vi "Configure Program Mode.vi"(0 "VISA resource name":refnum<visa-resource-name>, 1 "Voltage Low Limit (0 V)":dbl min=0.0 max=400.0 format="%.1f", 2 "Voltage High Limit (300 V)":dbl=300.0 min=0.0 max=400.0 format="%.1f", 3 "Single Step Mode (F:Disable)":bool, 5 "Loop Cycle (1)":i32=1 min=0 max=9999 step=1, 7 "Start Angle (0)":i32 min=0 max=359, 9 "End Angle: (0)":i32 min=0 max=359, 11 "error in (no error)":errorcluster, 12 "Frequency Low Limit (40 Hz)":dbl=45.0 min=0.0 max=500.0 format="%.1f", 13 "Frequency High Limit (500 Hz)":dbl=500.0 min=0.0 max=500.0 format="%.1f", 14 "Enable Over Current Fold Back (F:Disable)":bool) -> (4 "VISA resource name out":refnum<visa-resource-name>, 15 "error out":errorcluster)   [LabVIEW 2014, in "eec 6700.lvlib"]
doc: "Sets the instrument in program mode and configures the parameters in it.\n\nIn the program mode the instrument can be programmed for a sequence of operations/Settings with the help of a list of 50 sequential memories with 9 steps each. Each step can be configured with user configurable testing parameters such as test time, high and low limits, etc."
uses:
  <instrlib>/eec 6700/eec 6700.lvlib
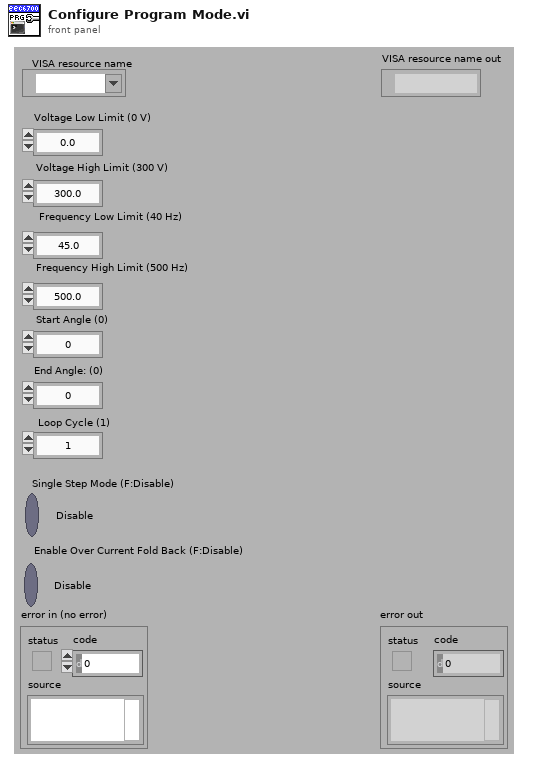
[diagram p1: front panel]
types:
  T1 = typedef "eec 6700.lvlib/Extended User Data.ctl" = cluster{"Firmware Version":string, "eec Models":enum16{"6605", "6610", "6620", "6630", "6650"}}
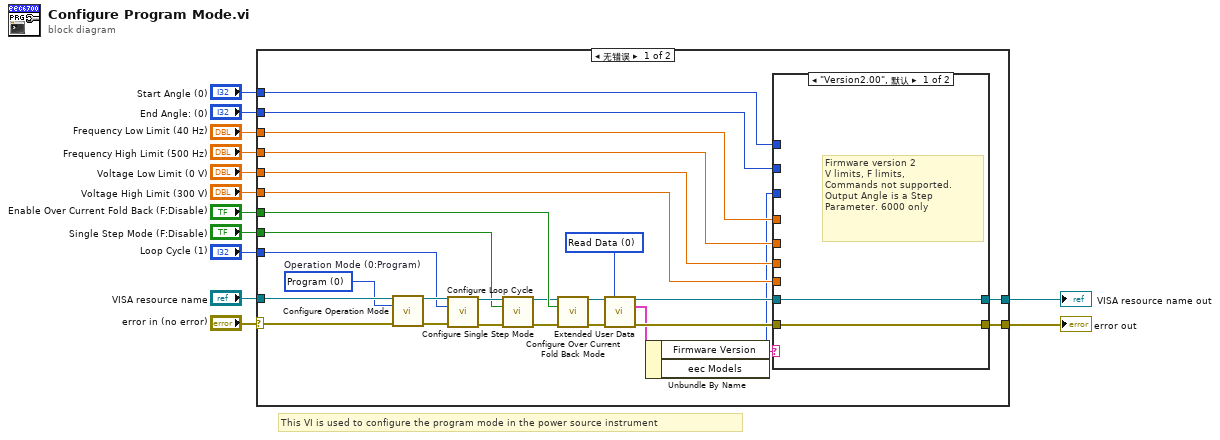
[diagram p0: block diagram]
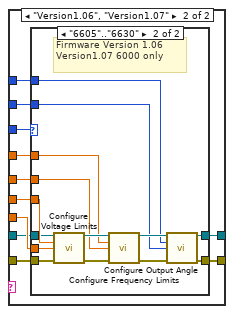
[diagram p2: hidden frame]
diagram:
  # "This VI is used to configure the program mode in the power source instrument"
  n1 = case shown="无错误" "error in (no error)" {
    selector: "error in (no error)" -> [w36 w72]
    tunnel: [w30 w72] -> w13
    tunnel: [w29 w71] -> w12
    tunnel: "VISA resource name" -> [w37 w71]
    tunnel: "Loop Cycle (1)" -> [w35 _]
    tunnel: "Single Step Mode (F:Disable)" -> [w34 _]
    tunnel: "Enable Over Current Fold Back (F:Disable)" -> [w33 _]
    tunnel: "Voltage High Limit (300 V)" -> [w28 _]
    tunnel: "Voltage Low Limit (0 V)" -> [w27 _]
    tunnel: "Frequency Low Limit (40 Hz)" -> [w26 _]
    tunnel: "Frequency High Limit (500 Hz)" -> [w16 _]
    tunnel: "End Angle: (0)" -> [w25 _]
    tunnel: "Start Angle (0)" -> [w24 _]
    frame No Error {
      w18 = u16 0 items=["Read Data", "Write Data", "Clear Data", "Clear ALL Data"] ("Action")
      w23 = u16 0 items=["Program", "Manual"]  # Operation Mode (0:Program)
      n2 = call <instrlib>:"Configure Operation Mode.vi"("VISA resource name"=w37, "Operation Mode (0:Program)"=w23, "error in (no error)"=w36) -> ("VISA resource name out"=w38:refnum<visa-resource-name>, "error out"=w39:errorcluster)  [unwired: 11 in]
      n3 = call <instrlib>:"Configure Loop Cycle.vi"("VISA resource name"=w38, "Loop Cycle (1)"=w35, "error in (no error)"=w39) -> ("VISA resource name out"=w40:refnum<visa-resource-name>, "error out"=w41:errorcluster)  [unwired: 11 in]
      n4 = call <instrlib>:"Configure Single Step Mode.vi"("VISA resource name"=w40, "Single Step Mode (F:Disable)"=w34, "error in (no error)"=w41) -> ("VISA resource name out"=w32:refnum<visa-resource-name>, "error out"=w31:errorcluster)  [unwired: 11 in]
      n5 = call <instrlib>:"Configure Over Current Fold Back Mode.vi"("VISA resource name"=w32, "Enable Over Current Fold Back (F:Disable)"=w33, "error in (no error)"=w31) -> ("VISA resource name out"=w22:refnum<visa-resource-name>, "error out"=w19:errorcluster)  [unwired: 11 in]
      n6 = call <instrlib>:"Extended User Data.vi"("VISA resource name"=w22, "Action"=w18, "Error In (no error)"=w19) -> ("VISA resource name out"=w21:refnum<visa-resource-name>, "User Data Out"=w17:T1, "Error Out"=w20:errorcluster)  [unwired: 10 in]
      n7 = Unbundle By Name(w17) -> ("Firmware Version"=w15:string, "eec Models"=w14:enum16{"6605", "6610", "6620", "6630", "6650"})
      n8 = case shown="\"Version2.00\", 默认" w15 {
        tunnel: [w42 w54] -> w30
        tunnel: [w43 w53] -> w29
        tunnel: w28 -> [_ w52]
        tunnel: w27 -> [_ w51]
        tunnel: w26 -> [_ w50]
        tunnel: w16 -> [_ w49]
        tunnel: w25 -> [_ w48]
        tunnel: w24 -> [_ w47]
        tunnel: w21 -> [w43 w46]
        tunnel: w20 -> [w42 w45]
        tunnel: w14 -> [_ w44]
        frame "Version2.00", Default {
          # "Firmware version 2\nV limits, F limits,\nCommands not supported.\nOutput Angle is a Step\nParameter. 6000 only"
        }
        frame "Version1.06", "Version1.07" {
          n9 = case shown="\"6605\"..\"6630\"" w44 {
            tunnel: [w55 w66] -> w54
            tunnel: [w56 w65] -> w53
            tunnel: w52 -> [_ w64]
            tunnel: w51 -> [_ w63]
            tunnel: w50 -> [_ w62]
            tunnel: w49 -> [_ w61]
            tunnel: w48 -> [_ w60]
            tunnel: w47 -> [_ w59]
            tunnel: w46 -> [w56 w58]
            tunnel: w45 -> [w55 w57]
            frame Default {
            }
            frame "6605".."6630" {
              # "Firmware Version 1.06\nVersion1.07 6000 only"
              n10 = call <instrlib>:"Configure Voltage Limits.vi"("VISA resource name"=w58, "Voltage Low Limit (0 V)"=w63, "Voltage High Limit (300 V)"=w64, "error in (no error)"=w57) -> ("VISA resource name out"=w70:refnum<visa-resource-name>, "error out"=w69:errorcluster)  [unwired: 10 in]
              n11 = call <instrlib>:"Configure Frequency Limits.vi"("VISA resource name"=w70, "Frequency Low Limit (40 Hz)"=w62, "Frequency High Limit (500 Hz)"=w61, "error in (no error)"=w69) -> ("VISA resource name out"=w68:refnum<visa-resource-name>, "error out"=w67:errorcluster)  [unwired: 10 in]
              n12 = call <instrlib>:"Configure Output Angle.vi"("VISA resource name"=w68, "Start Angle (0)"=w59, "End Angle: (0)"=w60, "error in (no error)"=w67) -> ("VISA resource name out"=w65:refnum<visa-resource-name>, "error out"=w66:errorcluster)  [unwired: 10 in]
            }
          }
        }
      }
    }
    frame Error {
    }
  }
  "error out" <- w13
  "VISA resource name out" <- w12
